vi "Write DAT.vi"   [LabVIEW 2019, in "Data.DAT.lvclass"]
uses:
  Data.DAT.lvclass
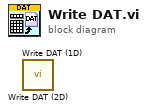
[diagram p0: block diagram]
diagram:
  n1 = call "Write DAT (2D).vi"() -> ()  [unwired: 10 in, 2 out]
  n2 = call "Write DAT (1D).vi"() -> ()  [unwired: 10 in, 2 out]
